vi "UART Write.vi"   [LabVIEW 2014, in "LMH-LINX.lvlib"]
uses:
  <vilib>/MakerHub/LINX/LMH-LINX.lvlib
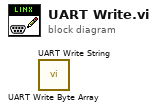
[diagram p0: block diagram]
diagram:
  n1 = call <vilib>:"UART Write Byte Array.vi"() -> ()  [unwired: 10 in, 2 out]
  n2 = call <vilib>:"UART Write String.vi"() -> ()  [unwired: 10 in, 2 out]
